vi "TestExec.Client, SW Items.vi"(7 "Module Q Name":string, 8 "error in":errorcluster, 10 "SW Items":T1[](array[typedef]), 11 "Q In":refnum<queue>) -> (0 "error out":errorcluster, 3 "Q Out":refnum<queue>)   [LabVIEW 2024]
uses:
  <vilib>/KATE/Queues/Q.Element.ctl
  Results/Result XML/TestResult.SW Item.ctl
  <vilib>/KATE/Queues/Queue Utils.lvlib
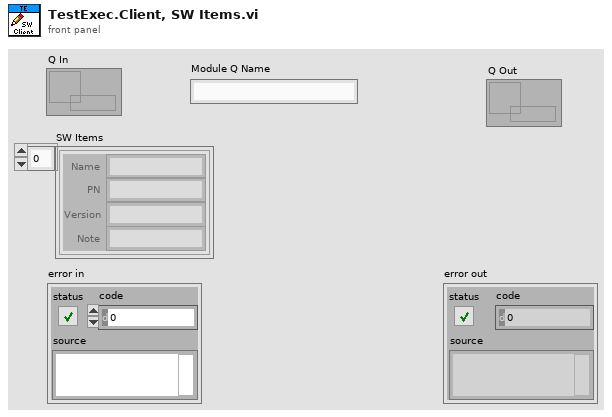
[diagram p1: front panel]
types:
  T1 = typedef "TestResult.SW Item.ctl" = cluster{"Name":string, "PN":string, "Version":string, "Note":string}
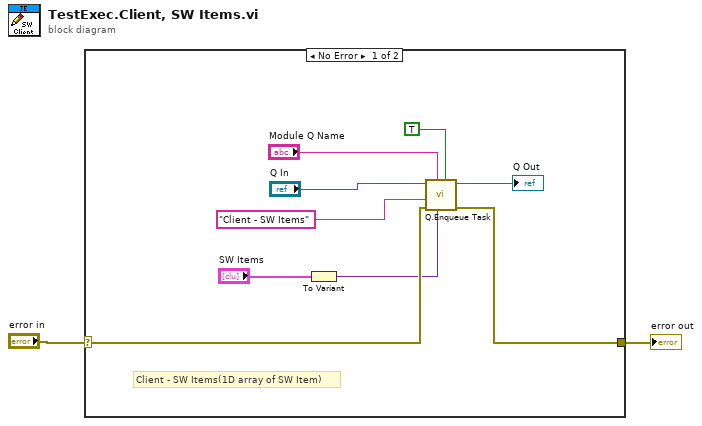
[diagram p0: block diagram]
diagram:
  n1 = case shown="No Error" "error in" {
    selector: "error in" -> [w8 w12]
    tunnel: [w9 w12] -> w1
    frame No Error {
      # "Client - SW Items(1D array of SW Item)"
      n2 = To Variant(anything="SW Items") -> (Variant=w7:variant)
      n3 = call <vilib>:"Q.Enqueue Task.vi"("Top of Q"=TRUE, "Data1"=w7, "Q Name"="Module Q Name", "Error In"=w8, "Task Name"="Client - SW Items" ("Cmd"), "Q In"="Q In") -> ("error out"=w9:errorcluster, "Q Out"=→"Q Out":refnum<queue>)  [unwired: 4 in]
    }
    frame Error {
    }
  }
  "error out" <- w1
